vi "Initialize Motors.vi"(0 "UniCyRO_Host_Sim in":refnum<class "UniCyRO_Host_Sim.lvclass">, 5 "Gyro Motor":refnum<class "DC Motor Controller.lvclass">, 7 "Drive Motor":refnum<class "DC Motor Controller.lvclass">, 9 "Torsion Motor":refnum<class "DC Motor Controller.lvclass">, 11 "error in (no error)":errorcluster, 12 "Gyro Motor Error":i32, 13 "Drive Motor Error":i32, 14 "Torsion Motor Error":i32) -> (4 "UniCyRO_Host_Sim out":refnum<class "UniCyRO_Host_Sim.lvclass">, 15 "error out":errorcluster)   [LabVIEW 2012, in "UniCyRO.lvlib" / "UniCyRO_Host_Sim.lvclass"]
uses:
  UniCyRO_Host_Sim.lvclass
  <instrlib>/DC Motor Controller/HAIOL/DC Motor Controller.lvclass
  UniCyRO_Host_Sim.lvclass/UniCyRO_Host_Sim.ctl
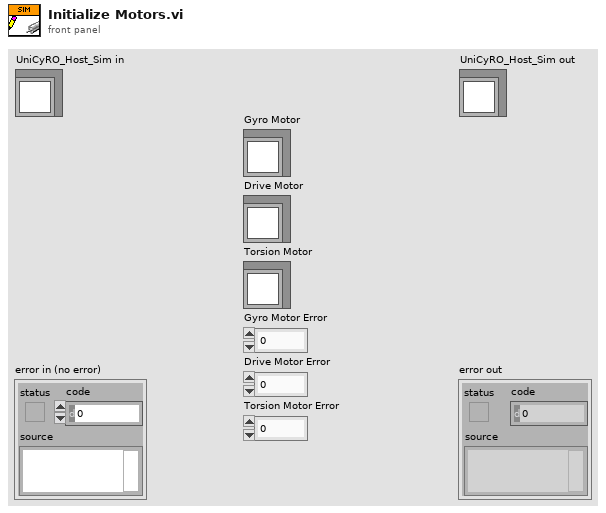
[diagram p1: front panel]
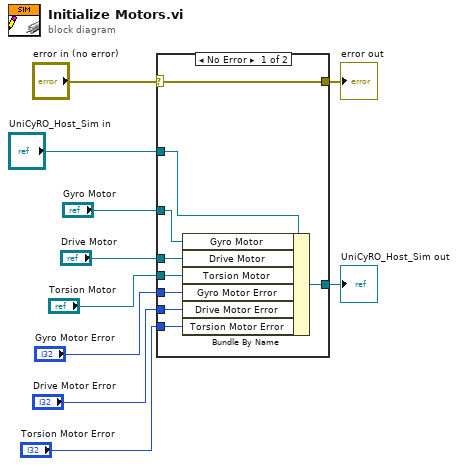
[diagram p0: block diagram]
diagram:
  n1 = case shown="No Error" "error in (no error)" {
    selector: "error in (no error)" -> [w19 w21]
    tunnel: [w19 w21] -> w9
    tunnel: [w17 w20] -> w7
    tunnel: "UniCyRO_Host_Sim in" -> [w18 w20]
    tunnel: "Gyro Motor" -> [w16 _]
    tunnel: "Drive Motor" -> [w15 _]
    tunnel: "Torsion Motor" -> [w14 _]
    tunnel: "Gyro Motor Error" -> [w13 _]
    tunnel: "Drive Motor Error" -> [w12 _]
    tunnel: "Torsion Motor Error" -> [w11 _]
    frame No Error {
      n2 = Bundle By Name(cluster=w18, "Gyro Motor"=w16, "Drive Motor"=w15, "Torsion Motor"=w14, "Gyro Motor Error"=w13, "Drive Motor Error"=w12, "Torsion Motor Error"=w11) -> (w17:refnum<class "UniCyRO_Host_Sim.lvclass">)
    }
    frame Error {
    }
  }
  "error out" <- w9
  "UniCyRO_Host_Sim out" <- w7
